vi "start_action.vi"(0 "HGF_ImaqDx":refnum<class "HGF_ImaqDx.lvclass">, 5 "error in (no error)":errorcluster) -> (14 "dup HGF_ImaqDx":refnum<class "HGF_ImaqDx.lvclass">, 19 "error out":errorcluster)   [LabVIEW 2014, in "HGF_IMAQ.lvlib" / "HGF_ImaqDx.lvclass"]
doc: "Starts an asynchronous acquisition that was previously configured with IMAQdx Configure Acquisition.vi. Use IMAQdx Stop Acquisition.vi to stop the acquisition."
uses:
  HGF_ImaqDx.lvclass
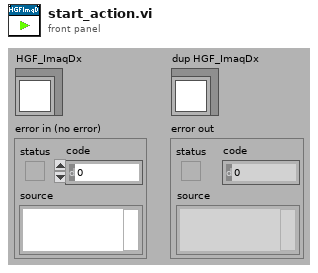
[diagram p1: front panel]
types:
  T1 = typedef "IMAQdx.ctl" = refnum<k21>
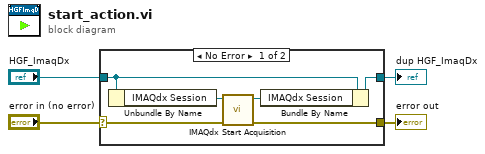
[diagram p0: block diagram]
diagram:
  n1 = case shown="No Error" "error in (no error)" {
    selector: "error in (no error)" -> [w5 w11]
    tunnel: "HGF_ImaqDx" -> [w9 w12]
    tunnel: [w7 w12] -> w3
    tunnel: [w6 w11] -> w2
    frame No Error {
      n2 = Unbundle By Name(w9) -> ("IMAQdx Session"=w10:T1)
      n3 = call <vilib>:"IMAQdx Start Acquisition.vi"("error in"=w5, "Session In"=w10) -> ("error out"=w6:errorcluster, "Session Out"=w8:T1)  [unwired: 8 out]
      n4 = Bundle By Name(cluster=w9, "IMAQdx Session"=w8) -> (w7:refnum<class "HGF_ImaqDx.lvclass">)
    }
    frame Error {
    }
  }
  "error out" <- w2
  "dup HGF_ImaqDx" <- w3
